vi "Pre Launch Init.vi"(11 "Coffee Shop in":refnum<class "Coffee Shop.lvclass">) -> (0 "error out":errorcluster, 3 "Coffee Shop out":refnum<class "Coffee Shop.lvclass">)   [LabVIEW 2023, in "Coffee Shop.lvlib" / "Coffee Shop.lvclass"]
doc: "(<B>Filename</B>: Actor Framework.lvlib:Actor.lvclass:Pre Launch Init.vi)\n\nDefines behavior that occurs after the Launch Nested Actor method is invoked but before the actor's Actor Core method begins running.\n\nBy default, this method does nothing. A descendant class may override it to define behavior."
uses:
  Coffee Shop.lvclass
  Table Data.ctl
  Entity Types.ctl
  Coffee Shop.lvclass/Coffee Shop.ctl
  <vilib>/ActorFramework/Actor/Actor.lvclass
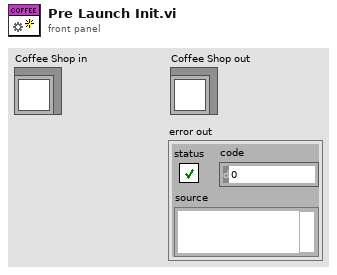
[diagram p1: front panel]
types:
  T1 = typedef "Coffee Shop.lvlib/Coffee Shop.lvclass/Table Data.ctl" = cluster{"Entity Type":T2, "Item Names":string[][]}
  T2 = typedef "Coffee Shop.lvlib/Coffee Shop.lvclass/Entity Types.ctl" = enum16{"Customer", "Cashier", "Barista"}
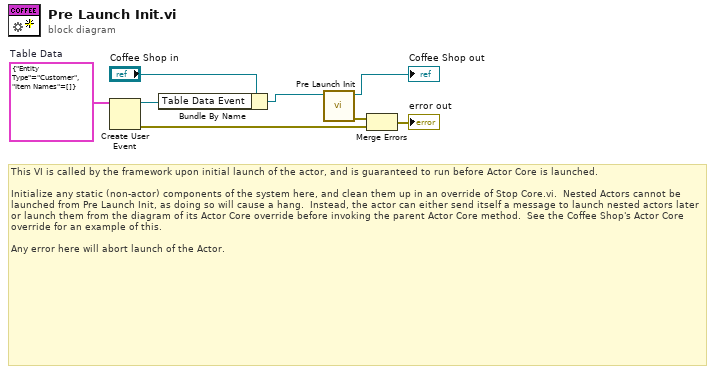
[diagram p0: block diagram]
diagram:
  w5 = T1 {"Entity Type"=enum."Customer", "Item Names"=[]}  # Table Data
  # "This VI is called by the framework upon initial launch of the actor, and is guaranteed to run before Actor Core is launched.\n\nInitialize any static (non-actor) components of the system here, and clean them up in an override of Stop Core.vi.  Nested Actors cannot be launched from Pre Launch Init, as doing so will cause a hang.  Instead, the actor can either send itself a message to launch nested actors later or launch them from the diagram of its Actor Core override before invoking the parent Actor Core method.  See the Coffee Shop's Actor Core override for an example of this.\n\nAny error here will abort launch of the Actor."
  n1 = Create User Event(user event datatype=w5) -> (user event=w4:refnum<user-event>, error out=w2:errorcluster)  [unwired: 1 in]
  n2 = Bundle By Name(cluster="Coffee Shop in", "Table Data Event"=w4) -> (w1:refnum<class "Coffee Shop.lvclass">)
  n3 = call-parent "Pre Launch Init.vi"("Actor in"=w1) -> ("error out"=w7:errorcluster, "Actor out"=→"Coffee Shop out":refnum<class "Coffee Shop.lvclass">)  [unwired: 9 in]
  n4 = Merge Errors(w7, w2) -> (→"error out":errorcluster)
